vi "X410 ADC Read.vi"() -> (3 "Data out":T1[](array[typedef]))   [LabVIEW 2023]
uses:
  <instrlib>/_niInstr/DSP/v1/Shared/Public/IQ Data.ctl
  <vilib>/rvi/eio/common/nirviEmuTemplateMethod_errors.vi
  <instrlib>/_niInstr/DSP/v1/FPGA/Public/Sub VIs/Data Conversion/I16 to IQ - 1 spc - S18.1.vi
  <vilib>/eio/EIONode/EIONode.xnode
  <instrlib>/_niInstr/DSP/v1/FPGA/niInstr DSP v1 FPGA.lvlib
  <instrlib>/_niInstr/DSP/v1/Shared/niInstr DSP v1 Shared.lvlib
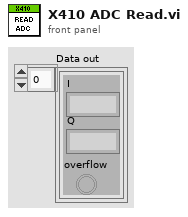
[diagram p1: front panel]
types:
  T1 = typedef "niInstr DSP v1 Shared.lvlib/IQ Data.ctl" = cluster{"I":fxp<+/-,18,1>, "Q":fxp<+/-,18,1>, "overflow":bool}
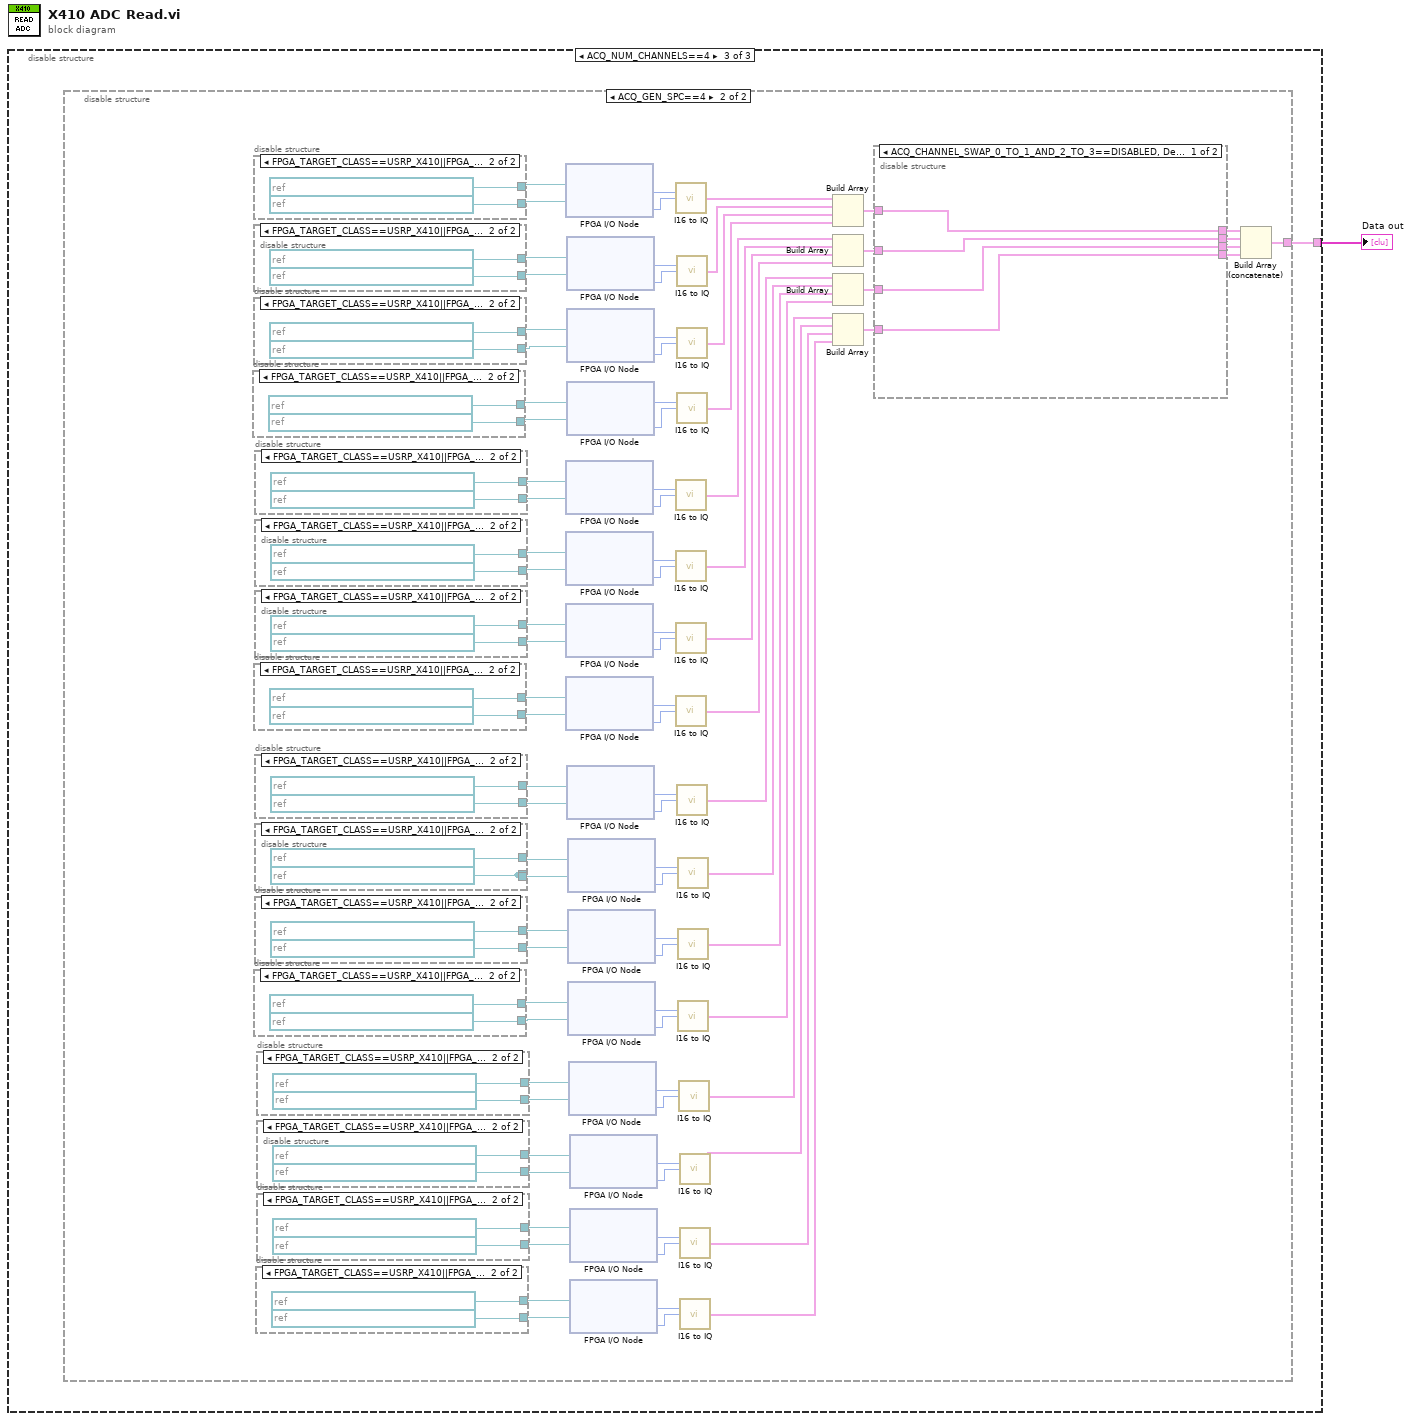
[diagram p0: block diagram]
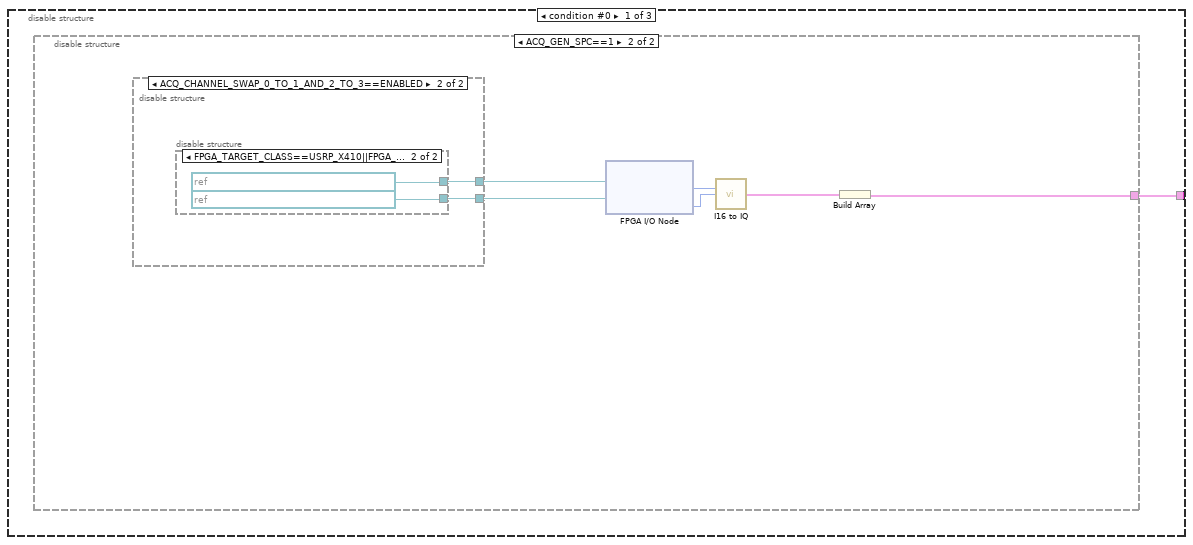
[diagram p2: hidden frame]
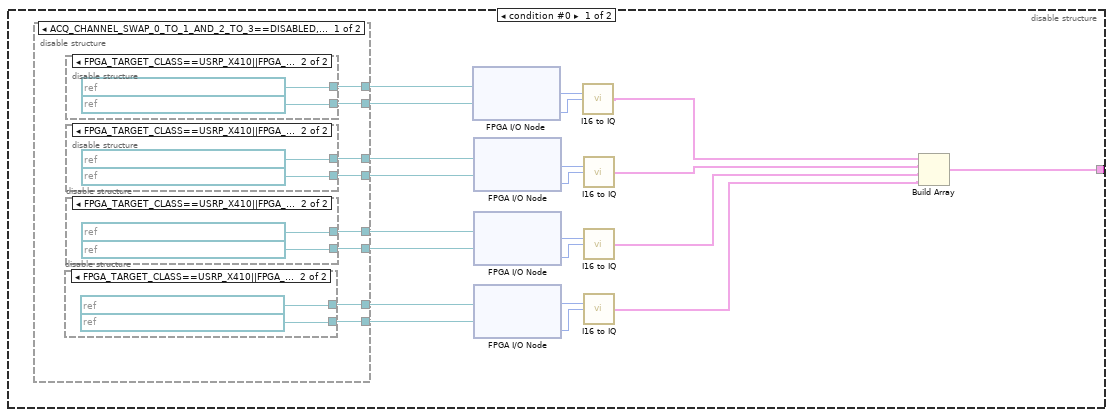
[diagram p3: hidden frame]
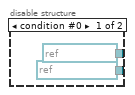
[diagram p4: hidden frame]
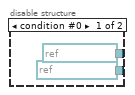
[diagram p5: hidden frame]
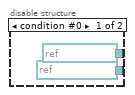
[diagram p6: hidden frame]
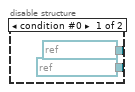
[diagram p7: hidden frame]
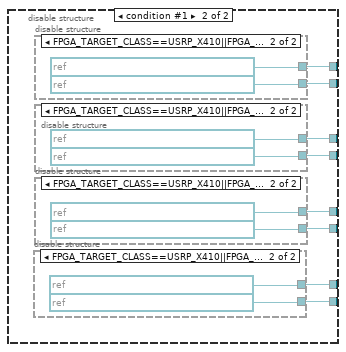
[diagram p8: hidden frame]
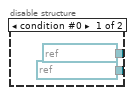
[diagram p9: hidden frame]
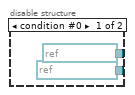
[diagram p10: hidden frame]
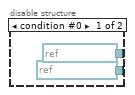
[diagram p11: hidden frame]
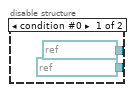
[diagram p12: hidden frame]
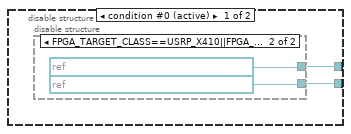
[diagram p13: hidden frame]
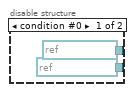
[diagram p14: hidden frame]
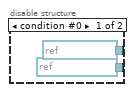
[diagram p15: hidden frame]
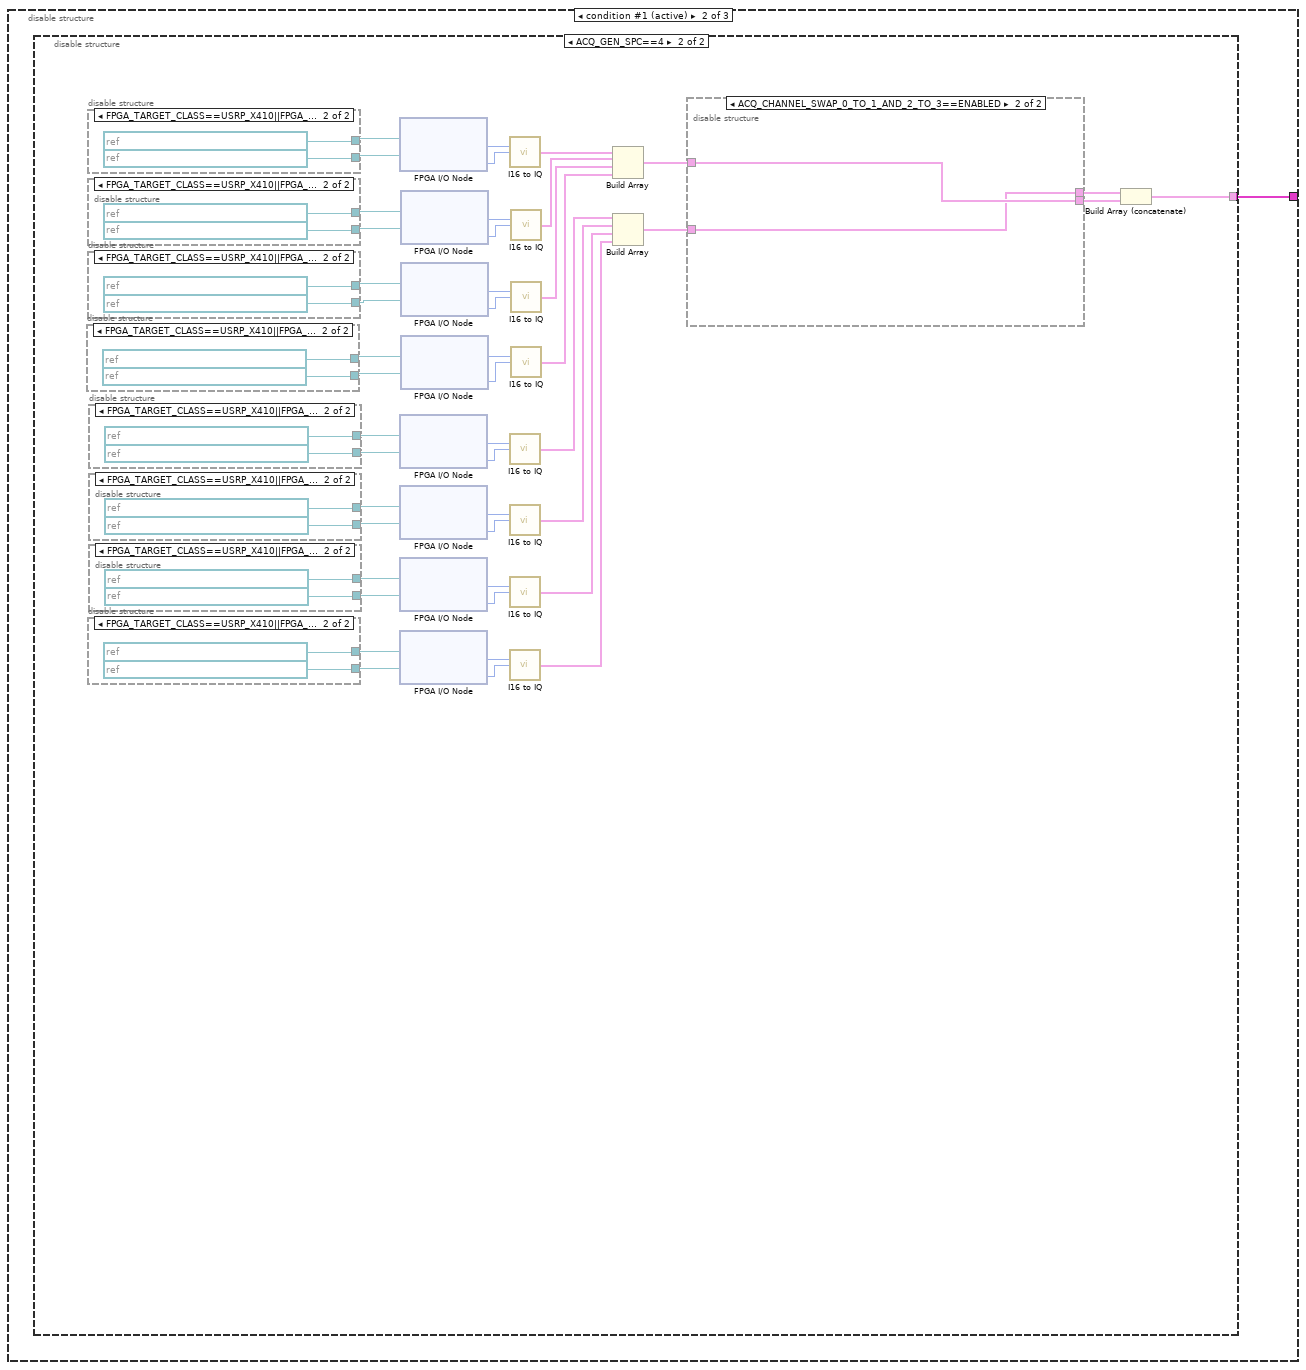
[diagram p16: hidden frame]
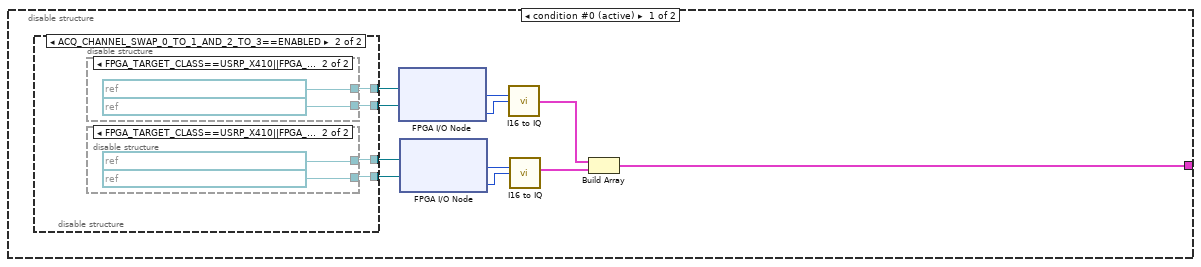
[diagram p17: hidden frame]
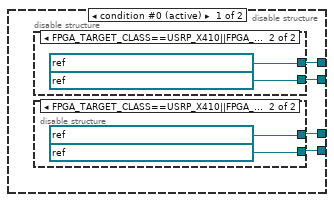
[diagram p18: hidden frame]
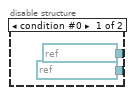
[diagram p19: hidden frame]
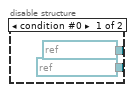
[diagram p20: hidden frame]
diagram:
  n1 = disable-structure shown="ACQ_NUM_CHANNELS==4" {
    disable-tunnel: [w2 w90 w207] -> w1
    frame condition #0 {
      n2 = disable-structure shown="ACQ_GEN_SPC==1" {
        disable-tunnel: [w15 w77] -> w2
        frame condition #0 {
          n3 = disable-structure shown="ACQ_CHANNEL_SWAP_0_TO_1_AND_2_TO_3==DISABLED, Default" {
            disable-tunnel: [w31 w55] -> w10
            disable-tunnel: [w30 w54] -> w9
            disable-tunnel: [w29 w53] -> w8
            disable-tunnel: [w28 w52] -> w7
            disable-tunnel: [w27 w51] -> w6
            disable-tunnel: [w26 w50] -> w5
            disable-tunnel: [w25 w49] -> w4
            disable-tunnel: [w24 w48] -> w3
            frame condition #0 (active) {
              n4 = disable-structure shown="FPGA_TARGET_CLASS==USRP_X410||FPGA_TARGET_CLASS==USRP_X410__EMBEDDED____UNSUPPORTED" {
                disable-tunnel: [refnum<k21> "RF 0/Rx/Q" ("FPGA I/O In") refnum<k21> "Daughterboard 0\\RF 0.Rx.Q3" ("FPGA I/O In")] -> w24
                disable-tunnel: [refnum<k21> "RF 0/Rx/I" ("FPGA I/O In") refnum<k21> "Daughterboard 0\\RF 0.Rx.I3" ("FPGA I/O In")] -> w25
                frame condition #0 {
                }
                frame condition #1 (active) {
                }
              }
              n5 = disable-structure shown="FPGA_TARGET_CLASS==USRP_X410||FPGA_TARGET_CLASS==USRP_X410__EMBEDDED____UNSUPPORTED" {
                disable-tunnel: [refnum<k21> "RF 0/Rx/Q" ("FPGA I/O In") refnum<k21> "Daughterboard 0\\RF 0.Rx.Q0" ("FPGA I/O In")] -> w30
                disable-tunnel: [refnum<k21> "RF 0/Rx/I" ("FPGA I/O In") refnum<k21> "Daughterboard 0\\RF 0.Rx.I0" ("FPGA I/O In")] -> w31
                frame condition #0 {
                }
                frame condition #1 (active) {
                }
              }
              n6 = disable-structure shown="FPGA_TARGET_CLASS==USRP_X410||FPGA_TARGET_CLASS==USRP_X410__EMBEDDED____UNSUPPORTED" {
                disable-tunnel: [refnum<k21> "RF 0/Rx/Q" ("FPGA I/O In") refnum<k21> "Daughterboard 0\\RF 0.Rx.Q1" ("FPGA I/O In")] -> w28
                disable-tunnel: [refnum<k21> "RF 0/Rx/I" ("FPGA I/O In") refnum<k21> "Daughterboard 0\\RF 0.Rx.I1" ("FPGA I/O In")] -> w29
                frame condition #0 {
                }
                frame condition #1 (active) {
                }
              }
              n7 = disable-structure shown="FPGA_TARGET_CLASS==USRP_X410||FPGA_TARGET_CLASS==USRP_X410__EMBEDDED____UNSUPPORTED" {
                disable-tunnel: [refnum<k21> "RF 0/Rx/Q" ("FPGA I/O In") refnum<k21> "Daughterboard 0\\RF 0.Rx.Q2" ("FPGA I/O In")] -> w26
                disable-tunnel: [refnum<k21> "RF 0/Rx/I" ("FPGA I/O In") refnum<k21> "Daughterboard 0\\RF 0.Rx.I2" ("FPGA I/O In")] -> w27
                frame condition #0 {
                }
                frame condition #1 (active) {
                }
              }
            }
            frame condition #1 {
              n8 = disable-structure shown="FPGA_TARGET_CLASS==USRP_X410||FPGA_TARGET_CLASS==USRP_X410__EMBEDDED____UNSUPPORTED" {
                disable-tunnel: [refnum<k21> "RF 0/Rx/Q" ("FPGA I/O In") refnum<k21> "Daughterboard 0\\Ch1RxDataQ3" ("FPGA I/O In")] -> w48
                disable-tunnel: [refnum<k21> "RF 0/Rx/I" ("FPGA I/O In") refnum<k21> "Daughterboard 0\\Ch1RxDataI3" ("FPGA I/O In")] -> w49
                frame condition #0 {
                }
                frame condition #1 (active) {
                }
              }
              n9 = disable-structure shown="FPGA_TARGET_CLASS==USRP_X410||FPGA_TARGET_CLASS==USRP_X410__EMBEDDED____UNSUPPORTED" {
                disable-tunnel: [refnum<k21> "RF 0/Rx/Q" ("FPGA I/O In") refnum<k21> "Daughterboard 0\\Ch1RxDataQ0" ("FPGA I/O In")] -> w54
                disable-tunnel: [refnum<k21> "RF 0/Rx/I" ("FPGA I/O In") refnum<k21> "Daughterboard 0\\Ch1RxDataI0" ("FPGA I/O In")] -> w55
                frame condition #0 {
                }
                frame condition #1 (active) {
                }
              }
              n10 = disable-structure shown="FPGA_TARGET_CLASS==USRP_X410||FPGA_TARGET_CLASS==USRP_X410__EMBEDDED____UNSUPPORTED" {
                disable-tunnel: [refnum<k21> "RF 0/Rx/Q" ("FPGA I/O In") refnum<k21> "Daughterboard 0\\Ch1RxDataQ1" ("FPGA I/O In")] -> w52
                disable-tunnel: [refnum<k21> "RF 0/Rx/I" ("FPGA I/O In") refnum<k21> "Daughterboard 0\\Ch1RxDataI1" ("FPGA I/O In")] -> w53
                frame condition #0 {
                }
                frame condition #1 (active) {
                }
              }
              n11 = disable-structure shown="FPGA_TARGET_CLASS==USRP_X410||FPGA_TARGET_CLASS==USRP_X410__EMBEDDED____UNSUPPORTED" {
                disable-tunnel: [refnum<k21> "RF 0/Rx/Q" ("FPGA I/O In") refnum<k21> "Daughterboard 0\\Ch1RxDataQ2" ("FPGA I/O In")] -> w50
                disable-tunnel: [refnum<k21> "RF 0/Rx/I" ("FPGA I/O In") refnum<k21> "Daughterboard 0\\Ch1RxDataI2" ("FPGA I/O In")] -> w51
                frame condition #0 {
                }
                frame condition #1 (active) {
                }
              }
            }
          }
          n12 = xnode "FPGA I/O Node"("FPGA I/O In"=w10, "FPGA I/O In"=w9) -> ("I/O Item"=w23:i16, "I/O Item"=w22:i16)  [unwired: 2 out]
          n13 = xnode "FPGA I/O Node"("FPGA I/O In"=w8, "FPGA I/O In"=w7) -> ("I/O Item"=w21:i16, "I/O Item"=w20:i16)  [unwired: 2 out]
          n14 = xnode "FPGA I/O Node"("FPGA I/O In"=w6, "FPGA I/O In"=w5) -> ("I/O Item"=w19:i16, "I/O Item"=w18:i16)  [unwired: 2 out]
          n15 = xnode "FPGA I/O Node"("FPGA I/O In"=w4, "FPGA I/O In"=w3) -> ("I/O Item"=w17:i16, "I/O Item"=w16:i16)  [unwired: 2 out]
          n16 = call-poly <instrlib>:"I16 to IQ.vi"("I"=w23, "Q"=w22) -> ("IQ"=w11:T1)  [unwired: 13 in]
          n17 = call-poly <instrlib>:"I16 to IQ.vi"("I"=w21, "Q"=w20) -> ("IQ"=w14:T1)  [unwired: 13 in]
          n18 = call-poly <instrlib>:"I16 to IQ.vi"("I"=w19, "Q"=w18) -> ("IQ"=w13:T1)  [unwired: 13 in]
          n19 = call-poly <instrlib>:"I16 to IQ.vi"("I"=w17, "Q"=w16) -> ("IQ"=w12:T1)  [unwired: 13 in]
          n20 = Build Array(w11, w14, w13, w12) -> (w15:T1[])
        }
        frame condition #1 (active) {
          n21 = disable-structure shown="ACQ_CHANNEL_SWAP_0_TO_1_AND_2_TO_3==ENABLED" {
            disable-tunnel: [w79 w85] -> w73
            disable-tunnel: [w78 w84] -> w72
            frame condition #0 (active) {
              n22 = disable-structure shown="FPGA_TARGET_CLASS==USRP_X410||FPGA_TARGET_CLASS==USRP_X410__EMBEDDED____UNSUPPORTED" {
                disable-tunnel: [refnum<k21> "RF 0/Rx/Q" ("FPGA I/O In") refnum<k21> "Daughterboard 0\\RF 0.Rx.Q" ("FPGA I/O In")] -> w78
                disable-tunnel: [refnum<k21> "RF 0/Rx/I" ("FPGA I/O In") refnum<k21> "Daughterboard 0\\RF 0.Rx.I" ("FPGA I/O In")] -> w79
                frame condition #0 {
                }
                frame condition #1 (active) {
                }
              }
            }
            frame condition #1 {
              n23 = disable-structure shown="FPGA_TARGET_CLASS==USRP_X410||FPGA_TARGET_CLASS==USRP_X410__EMBEDDED____UNSUPPORTED" {
                disable-tunnel: [refnum<k21> "RF 0/Rx/Q" ("FPGA I/O In") refnum<k21> "Daughterboard 0\\Ch1RxDataQ" ("FPGA I/O In")] -> w84
                disable-tunnel: [refnum<k21> "RF 0/Rx/I" ("FPGA I/O In") refnum<k21> "Daughterboard 0\\Ch1RxDataI" ("FPGA I/O In")] -> w85
                frame condition #0 {
                }
                frame condition #1 (active) {
                }
              }
            }
          }
          n24 = xnode "FPGA I/O Node"("FPGA I/O In"=w73, "FPGA I/O In"=w72) -> ("I/O Item"=w76:i16, "I/O Item"=w75:i16)  [unwired: 2 out]
          n25 = call-poly <instrlib>:"I16 to IQ.vi"("I"=w76, "Q"=w75) -> ("IQ"=w74:T1)  [unwired: 13 in]
          n26 = Build Array(w74) -> (w77:T1[])
        }
      }
    }
    frame condition #1 (active) {
      n27 = disable-structure shown="ACQ_GEN_SPC==4" {
        disable-tunnel: [w91 w170] -> w90
        frame condition #0 (active) {
          n28 = disable-structure shown="ACQ_CHANNEL_SWAP_0_TO_1_AND_2_TO_3==ENABLED" {
            disable-tunnel: [w105 w117] -> w97
            disable-tunnel: [w104 w116] -> w96
            disable-tunnel: [w103 w115] -> w95
            disable-tunnel: [w102 w114] -> w94
            frame condition #0 (active) {
              n29 = disable-structure shown="FPGA_TARGET_CLASS==USRP_X410||FPGA_TARGET_CLASS==USRP_X410__EMBEDDED____UNSUPPORTED" {
                disable-tunnel: [refnum<k21> "RF 0/Rx/Q" ("FPGA I/O In") refnum<k21> "Daughterboard 0\\RF 0.Rx.Q" ("FPGA I/O In")] -> w103
                disable-tunnel: [refnum<k21> "RF 0/Rx/I" ("FPGA I/O In") refnum<k21> "Daughterboard 0\\RF 0.Rx.I" ("FPGA I/O In")] -> w102
                frame condition #0 {
                }
                frame condition #1 (active) {
                }
              }
              n30 = disable-structure shown="FPGA_TARGET_CLASS==USRP_X410||FPGA_TARGET_CLASS==USRP_X410__EMBEDDED____UNSUPPORTED" {
                disable-tunnel: [refnum<k21> "RF 0/Rx/Q" ("FPGA I/O In") refnum<k21> "Daughterboard 0\\RF 1.Rx.Q" ("FPGA I/O In")] -> w105
                disable-tunnel: [refnum<k21> "RF 0/Rx/I" ("FPGA I/O In") refnum<k21> "Daughterboard 0\\RF 1.Rx.I" ("FPGA I/O In")] -> w104
                frame condition #0 {
                }
                frame condition #1 (active) {
                }
              }
            }
            frame condition #1 {
              n31 = disable-structure shown="FPGA_TARGET_CLASS==USRP_X410||FPGA_TARGET_CLASS==USRP_X410__EMBEDDED____UNSUPPORTED" {
                disable-tunnel: [refnum<k21> "RF 0/Rx/Q" ("FPGA I/O In") refnum<k21> "Daughterboard 0\\Ch1RxDataQ" ("FPGA I/O In")] -> w115
                disable-tunnel: [refnum<k21> "RF 0/Rx/I" ("FPGA I/O In") refnum<k21> "Daughterboard 0\\Ch1RxDataI" ("FPGA I/O In")] -> w114
                frame condition #0 {
                }
                frame condition #1 (active) {
                }
              }
              n32 = disable-structure shown="FPGA_TARGET_CLASS==USRP_X410||FPGA_TARGET_CLASS==USRP_X410__EMBEDDED____UNSUPPORTED" {
                disable-tunnel: [refnum<k21> "RF 0/Rx/Q" ("FPGA I/O In") refnum<k21> "Daughterboard 0\\Ch0RxDataQ" ("FPGA I/O In")] -> w117
                disable-tunnel: [refnum<k21> "RF 0/Rx/I" ("FPGA I/O In") refnum<k21> "Daughterboard 0\\Ch0RxDataI" ("FPGA I/O In")] -> w116
                frame condition #0 {
                }
                frame condition #1 (active) {
                }
              }
            }
          }
          n33 = xnode "FPGA I/O Node"("FPGA I/O In"=w94, "FPGA I/O In"=w95) -> ("I/O Item"=w101:i16, "I/O Item"=w100:i16)  [unwired: 2 out]
          n34 = xnode "FPGA I/O Node"("FPGA I/O In"=w96, "FPGA I/O In"=w97) -> ("I/O Item"=w99:i16, "I/O Item"=w98:i16)  [unwired: 2 out]
          n35 = call-poly <instrlib>:"I16 to IQ.vi"("I"=w101, "Q"=w100) -> ("IQ"=w93:T1)  [unwired: 13 in]
          n36 = call-poly <instrlib>:"I16 to IQ.vi"("I"=w99, "Q"=w98) -> ("IQ"=w92:T1)  [unwired: 13 in]
          n37 = Build Array(w93, w92) -> (w91:T1[])
        }
        frame condition #1 {
          n38 = disable-structure shown="FPGA_TARGET_CLASS==USRP_X410||FPGA_TARGET_CLASS==USRP_X410__EMBEDDED____UNSUPPORTED" {
            disable-tunnel: [refnum<k21> "RF 0/Rx/Q" ("FPGA I/O In") refnum<k21> "Daughterboard 0\\RF 0.Rx.Q3" ("FPGA I/O In")] -> w145
            disable-tunnel: [refnum<k21> "RF 0/Rx/I" ("FPGA I/O In") refnum<k21> "Daughterboard 0\\RF 0.Rx.I3" ("FPGA I/O In")] -> w144
            frame condition #0 {
            }
            frame condition #1 (active) {
            }
          }
          n39 = disable-structure shown="FPGA_TARGET_CLASS==USRP_X410||FPGA_TARGET_CLASS==USRP_X410__EMBEDDED____UNSUPPORTED" {
            disable-tunnel: [refnum<k21> "RF 0/Rx/Q" ("FPGA I/O In") refnum<k21> "Daughterboard 0\\RF 0.Rx.Q0" ("FPGA I/O In")] -> w139
            disable-tunnel: [refnum<k21> "RF 0/Rx/I" ("FPGA I/O In") refnum<k21> "Daughterboard 0\\RF 0.Rx.I0" ("FPGA I/O In")] -> w138
            frame condition #0 {
            }
            frame condition #1 (active) {
            }
          }
          n40 = disable-structure shown="FPGA_TARGET_CLASS==USRP_X410||FPGA_TARGET_CLASS==USRP_X410__EMBEDDED____UNSUPPORTED" {
            disable-tunnel: [refnum<k21> "RF 0/Rx/Q" ("FPGA I/O In") refnum<k21> "Daughterboard 0\\RF 0.Rx.Q1" ("FPGA I/O In")] -> w141
            disable-tunnel: [refnum<k21> "RF 0/Rx/I" ("FPGA I/O In") refnum<k21> "Daughterboard 0\\RF 0.Rx.I1" ("FPGA I/O In")] -> w140
            frame condition #0 {
            }
            frame condition #1 (active) {
            }
          }
          n41 = disable-structure shown="FPGA_TARGET_CLASS==USRP_X410||FPGA_TARGET_CLASS==USRP_X410__EMBEDDED____UNSUPPORTED" {
            disable-tunnel: [refnum<k21> "RF 0/Rx/Q" ("FPGA I/O In") refnum<k21> "Daughterboard 0\\RF 0.Rx.Q2" ("FPGA I/O In")] -> w143
            disable-tunnel: [refnum<k21> "RF 0/Rx/I" ("FPGA I/O In") refnum<k21> "Daughterboard 0\\RF 0.Rx.I2" ("FPGA I/O In")] -> w142
            frame condition #0 {
            }
            frame condition #1 (active) {
            }
          }
          n42 = disable-structure shown="FPGA_TARGET_CLASS==USRP_X410||FPGA_TARGET_CLASS==USRP_X410__EMBEDDED____UNSUPPORTED" {
            disable-tunnel: [refnum<k21> "RF 0/Rx/Q" ("FPGA I/O In") refnum<k21> "Daughterboard 0\\RF 1.Rx.Q3" ("FPGA I/O In")] -> w153
            disable-tunnel: [refnum<k21> "RF 0/Rx/I" ("FPGA I/O In") refnum<k21> "Daughterboard 0\\RF 1.Rx.I3" ("FPGA I/O In")] -> w152
            frame condition #0 {
            }
            frame condition #1 (active) {
            }
          }
          n43 = disable-structure shown="FPGA_TARGET_CLASS==USRP_X410||FPGA_TARGET_CLASS==USRP_X410__EMBEDDED____UNSUPPORTED" {
            disable-tunnel: [refnum<k21> "RF 0/Rx/Q" ("FPGA I/O In") refnum<k21> "Daughterboard 0\\RF 1.Rx.Q0" ("FPGA I/O In")] -> w147
            disable-tunnel: [refnum<k21> "RF 0/Rx/I" ("FPGA I/O In") refnum<k21> "Daughterboard 0\\RF 1.Rx.I0" ("FPGA I/O In")] -> w146
            frame condition #0 {
            }
            frame condition #1 (active) {
            }
          }
          n44 = disable-structure shown="FPGA_TARGET_CLASS==USRP_X410||FPGA_TARGET_CLASS==USRP_X410__EMBEDDED____UNSUPPORTED" {
            disable-tunnel: [refnum<k21> "RF 0/Rx/Q" ("FPGA I/O In") refnum<k21> "Daughterboard 0\\RF 1.Rx.Q1" ("FPGA I/O In")] -> w149
            disable-tunnel: [refnum<k21> "RF 0/Rx/I" ("FPGA I/O In") refnum<k21> "Daughterboard 0\\RF 1.Rx.I1" ("FPGA I/O In")] -> w148
            frame condition #0 {
            }
            frame condition #1 (active) {
            }
          }
          n45 = disable-structure shown="FPGA_TARGET_CLASS==USRP_X410||FPGA_TARGET_CLASS==USRP_X410__EMBEDDED____UNSUPPORTED" {
            disable-tunnel: [refnum<k21> "RF 0/Rx/Q" ("FPGA I/O In") refnum<k21> "Daughterboard 0\\RF 1.Rx.Q2" ("FPGA I/O In")] -> w151
            disable-tunnel: [refnum<k21> "RF 0/Rx/I" ("FPGA I/O In") refnum<k21> "Daughterboard 0\\RF 1.Rx.I2" ("FPGA I/O In")] -> w150
            frame condition #0 {
            }
            frame condition #1 (active) {
            }
          }
          n46 = xnode "FPGA I/O Node"("FPGA I/O In"=w138, "FPGA I/O In"=w139) -> ("I/O Item"=w169:i16, "I/O Item"=w168:i16)  [unwired: 2 out]
          n47 = xnode "FPGA I/O Node"("FPGA I/O In"=w146, "FPGA I/O In"=w147) -> ("I/O Item"=w161:i16, "I/O Item"=w160:i16)  [unwired: 2 out]
          n48 = xnode "FPGA I/O Node"("FPGA I/O In"=w148, "FPGA I/O In"=w149) -> ("I/O Item"=w159:i16, "I/O Item"=w158:i16)  [unwired: 2 out]
          n49 = xnode "FPGA I/O Node"("FPGA I/O In"=w150, "FPGA I/O In"=w151) -> ("I/O Item"=w157:i16, "I/O Item"=w156:i16)  [unwired: 2 out]
          n50 = xnode "FPGA I/O Node"("FPGA I/O In"=w152, "FPGA I/O In"=w153) -> ("I/O Item"=w155:i16, "I/O Item"=w154:i16)  [unwired: 2 out]
          n51 = xnode "FPGA I/O Node"("FPGA I/O In"=w140, "FPGA I/O In"=w141) -> ("I/O Item"=w167:i16, "I/O Item"=w166:i16)  [unwired: 2 out]
          n52 = xnode "FPGA I/O Node"("FPGA I/O In"=w142, "FPGA I/O In"=w143) -> ("I/O Item"=w165:i16, "I/O Item"=w164:i16)  [unwired: 2 out]
          n53 = xnode "FPGA I/O Node"("FPGA I/O In"=w144, "FPGA I/O In"=w145) -> ("I/O Item"=w163:i16, "I/O Item"=w162:i16)  [unwired: 2 out]
          n54 = call-poly <instrlib>:"I16 to IQ.vi"("I"=w169, "Q"=w168) -> ("IQ"=w137:T1)  [unwired: 13 in]
          n55 = call-poly <instrlib>:"I16 to IQ.vi"("I"=w161, "Q"=w160) -> ("IQ"=w133:T1)  [unwired: 13 in]
          n56 = call-poly <instrlib>:"I16 to IQ.vi"("I"=w159, "Q"=w158) -> ("IQ"=w132:T1)  [unwired: 13 in]
          n57 = call-poly <instrlib>:"I16 to IQ.vi"("I"=w157, "Q"=w156) -> ("IQ"=w131:T1)  [unwired: 13 in]
          n58 = call-poly <instrlib>:"I16 to IQ.vi"("I"=w155, "Q"=w154) -> ("IQ"=w130:T1)  [unwired: 13 in]
          n59 = call-poly <instrlib>:"I16 to IQ.vi"("I"=w167, "Q"=w166) -> ("IQ"=w136:T1)  [unwired: 13 in]
          n60 = call-poly <instrlib>:"I16 to IQ.vi"("I"=w165, "Q"=w164) -> ("IQ"=w135:T1)  [unwired: 13 in]
          n61 = call-poly <instrlib>:"I16 to IQ.vi"("I"=w163, "Q"=w162) -> ("IQ"=w134:T1)  [unwired: 13 in]
          n62 = Build Array(w137, w136, w135, w134) -> (w129:T1[])
          n63 = Build Array(w133, w132, w131, w130) -> (w127:T1[])
          n64 = disable-structure shown="ACQ_CHANNEL_SWAP_0_TO_1_AND_2_TO_3==ENABLED" {
            disable-tunnel: w129 -> [w172 w174]
            disable-tunnel: [w172 w173] -> w128
            disable-tunnel: [w171 w174] -> w126
            disable-tunnel: w127 -> [w171 w173]
            frame condition #0 (active) {
            }
            frame condition #1 {
            }
          }
          n65 = Build Array (concatenate)(w128, w126) -> (w170:T1[])
        }
      }
    }
    frame condition #2 {
      n66 = disable-structure shown="ACQ_GEN_SPC==4" {
        disable-tunnel: [w216 w345] -> w207
        frame condition #0 (active) {
          n67 = disable-structure shown="FPGA_TARGET_CLASS==USRP_X410||FPGA_TARGET_CLASS==USRP_X410__EMBEDDED____UNSUPPORTED" {
            disable-tunnel: [refnum<k21> "RF 0/Rx/Q" ("FPGA I/O In") refnum<k21> "Daughterboard 1\\RF 1.Rx.Q" ("FPGA I/O In")] -> w224
            disable-tunnel: [refnum<k21> "RF 0/Rx/I" ("FPGA I/O In") refnum<k21> "Daughterboard 1\\RF 1.Rx.I" ("FPGA I/O In")] -> w223
            frame condition #0 {
            }
            frame condition #1 (active) {
            }
          }
          n68 = disable-structure shown="FPGA_TARGET_CLASS==USRP_X410||FPGA_TARGET_CLASS==USRP_X410__EMBEDDED____UNSUPPORTED" {
            disable-tunnel: [refnum<k21> "RF 0/Rx/Q" ("FPGA I/O In") refnum<k21> "Daughterboard 0\\RF 0.Rx.Q" ("FPGA I/O In")] -> w218
            disable-tunnel: [refnum<k21> "RF 0/Rx/I" ("FPGA I/O In") refnum<k21> "Daughterboard 0\\RF 0.Rx.I" ("FPGA I/O In")] -> w217
            frame condition #0 {
            }
            frame condition #1 (active) {
            }
          }
          n69 = disable-structure shown="FPGA_TARGET_CLASS==USRP_X410||FPGA_TARGET_CLASS==USRP_X410__EMBEDDED____UNSUPPORTED" {
            disable-tunnel: [refnum<k21> "RF 0/Rx/Q" ("FPGA I/O In") refnum<k21> "Daughterboard 0\\RF 1.Rx.Q" ("FPGA I/O In")] -> w220
            disable-tunnel: [refnum<k21> "RF 0/Rx/I" ("FPGA I/O In") refnum<k21> "Daughterboard 0\\RF 1.Rx.I" ("FPGA I/O In")] -> w219
            frame condition #0 {
            }
            frame condition #1 (active) {
            }
          }
          n70 = disable-structure shown="FPGA_TARGET_CLASS==USRP_X410||FPGA_TARGET_CLASS==USRP_X410__EMBEDDED____UNSUPPORTED" {
            disable-tunnel: [refnum<k21> "RF 0/Rx/Q" ("FPGA I/O In") refnum<k21> "Daughterboard 1\\RF 0.Rx.Q" ("FPGA I/O In")] -> w222
            disable-tunnel: [refnum<k21> "RF 0/Rx/I" ("FPGA I/O In") refnum<k21> "Daughterboard 1\\RF 0.Rx.I" ("FPGA I/O In")] -> w221
            frame condition #0 {
            }
            frame condition #1 (active) {
            }
          }
          n71 = xnode "FPGA I/O Node"("FPGA I/O In"=w217, "FPGA I/O In"=w218) -> ("I/O Item"=w232:i16, "I/O Item"=w231:i16)  [unwired: 2 out]
          n72 = xnode "FPGA I/O Node"("FPGA I/O In"=w219, "FPGA I/O In"=w220) -> ("I/O Item"=w230:i16, "I/O Item"=w229:i16)  [unwired: 2 out]
          n73 = xnode "FPGA I/O Node"("FPGA I/O In"=w221, "FPGA I/O In"=w222) -> ("I/O Item"=w228:i16, "I/O Item"=w227:i16)  [unwired: 2 out]
          n74 = xnode "FPGA I/O Node"("FPGA I/O In"=w223, "FPGA I/O In"=w224) -> ("I/O Item"=w226:i16, "I/O Item"=w225:i16)  [unwired: 2 out]
          n75 = call-poly <instrlib>:"I16 to IQ.vi"("I"=w232, "Q"=w231) -> ("IQ"=w215:T1)  [unwired: 13 in]
          n76 = call-poly <instrlib>:"I16 to IQ.vi"("I"=w230, "Q"=w229) -> ("IQ"=w210:T1)  [unwired: 13 in]
          n77 = call-poly <instrlib>:"I16 to IQ.vi"("I"=w228, "Q"=w227) -> ("IQ"=w209:T1)  [unwired: 13 in]
          n78 = call-poly <instrlib>:"I16 to IQ.vi"("I"=w226, "Q"=w225) -> ("IQ"=w208:T1)  [unwired: 13 in]
          n79 = disable-structure shown="ACQ_CHANNEL_SWAP_0_TO_1_AND_2_TO_3==ENABLED" {
            disable-tunnel: w215 -> [w235 w239]
            disable-tunnel: [w236 w239] -> w213
            disable-tunnel: w210 -> [w236 w240]
            disable-tunnel: [w235 w240] -> w214
            disable-tunnel: [w234 w238] -> w212
            disable-tunnel: w209 -> [w234 w237]
            disable-tunnel: [w233 w237] -> w211
            disable-tunnel: w208 -> [w233 w238]
            frame condition #0 (active) {
            }
            frame condition #1 {
            }
          }
          n80 = Build Array(w214, w213, w212, w211) -> (w216:T1[])
        }
        frame condition #1 {
          n81 = disable-structure shown="FPGA_TARGET_CLASS==USRP_X410||FPGA_TARGET_CLASS==USRP_X410__EMBEDDED____UNSUPPORTED" {
            disable-tunnel: [refnum<k21> "RF 0/Rx/Q" ("FPGA I/O In") refnum<k21> "Daughterboard 0\\RF 0.Rx.Q3" ("FPGA I/O In")] -> w288
            disable-tunnel: [refnum<k21> "RF 0/Rx/I" ("FPGA I/O In") refnum<k21> "Daughterboard 0\\RF 0.Rx.I3" ("FPGA I/O In")] -> w287
            frame condition #0 {
            }
            frame condition #1 (active) {
            }
          }
          n82 = disable-structure shown="FPGA_TARGET_CLASS==USRP_X410||FPGA_TARGET_CLASS==USRP_X410__EMBEDDED____UNSUPPORTED" {
            disable-tunnel: [refnum<k21> "RF 0/Rx/Q" ("FPGA I/O In") refnum<k21> "Daughterboard 0\\RF 0.Rx.Q0" ("FPGA I/O In")] -> w282
            disable-tunnel: [refnum<k21> "RF 0/Rx/I" ("FPGA I/O In") refnum<k21> "Daughterboard 0\\RF 0.Rx.I0" ("FPGA I/O In")] -> w281
            frame condition #0 {
            }
            frame condition #1 (active) {
            }
          }
          n83 = disable-structure shown="FPGA_TARGET_CLASS==USRP_X410||FPGA_TARGET_CLASS==USRP_X410__EMBEDDED____UNSUPPORTED" {
            disable-tunnel: [refnum<k21> "RF 0/Rx/Q" ("FPGA I/O In") refnum<k21> "Daughterboard 0\\RF 0.Rx.Q1" ("FPGA I/O In")] -> w284
            disable-tunnel: [refnum<k21> "RF 0/Rx/I" ("FPGA I/O In") refnum<k21> "Daughterboard 0\\RF 0.Rx.I1" ("FPGA I/O In")] -> w283
            frame condition #0 {
            }
            frame condition #1 (active) {
            }
          }
          n84 = disable-structure shown="FPGA_TARGET_CLASS==USRP_X410||FPGA_TARGET_CLASS==USRP_X410__EMBEDDED____UNSUPPORTED" {
            disable-tunnel: [refnum<k21> "RF 0/Rx/Q" ("FPGA I/O In") refnum<k21> "Daughterboard 0\\RF 0.Rx.Q2" ("FPGA I/O In")] -> w286
            disable-tunnel: [refnum<k21> "RF 0/Rx/I" ("FPGA I/O In") refnum<k21> "Daughterboard 0\\RF 0.Rx.I2" ("FPGA I/O In")] -> w285
            frame condition #0 {
            }
            frame condition #1 (active) {
            }
          }
          n85 = disable-structure shown="FPGA_TARGET_CLASS==USRP_X410||FPGA_TARGET_CLASS==USRP_X410__EMBEDDED____UNSUPPORTED" {
            disable-tunnel: [refnum<k21> "RF 0/Rx/Q" ("FPGA I/O In") refnum<k21> "Daughterboard 0\\RF 1.Rx.Q3" ("FPGA I/O In")] -> w296
            disable-tunnel: [refnum<k21> "RF 0/Rx/I" ("FPGA I/O In") refnum<k21> "Daughterboard 0\\RF 1.Rx.I3" ("FPGA I/O In")] -> w295
            frame condition #0 {
            }
            frame condition #1 (active) {
            }
          }
          n86 = disable-structure shown="FPGA_TARGET_CLASS==USRP_X410||FPGA_TARGET_CLASS==USRP_X410__EMBEDDED____UNSUPPORTED" {
            disable-tunnel: [refnum<k21> "RF 0/Rx/Q" ("FPGA I/O In") refnum<k21> "Daughterboard 1\\RF 0.Rx.Q3" ("FPGA I/O In")] -> w304
            disable-tunnel: [refnum<k21> "RF 0/Rx/I" ("FPGA I/O In") refnum<k21> "Daughterboard 1\\RF 0.Rx.I3" ("FPGA I/O In")] -> w303
            frame condition #0 {
            }
            frame condition #1 (active) {
            }
          }
          n87 = disable-structure shown="FPGA_TARGET_CLASS==USRP_X410||FPGA_TARGET_CLASS==USRP_X410__EMBEDDED____UNSUPPORTED" {
            disable-tunnel: [refnum<k21> "RF 0/Rx/Q" ("FPGA I/O In") refnum<k21> "Daughterboard 0\\RF 1.Rx.Q0" ("FPGA I/O In")] -> w290
            disable-tunnel: [refnum<k21> "RF 0/Rx/I" ("FPGA I/O In") refnum<k21> "Daughterboard 0\\RF 1.Rx.I0" ("FPGA I/O In")] -> w289
            frame condition #0 {
            }
            frame condition #1 (active) {
            }
          }
          n88 = disable-structure shown="FPGA_TARGET_CLASS==USRP_X410||FPGA_TARGET_CLASS==USRP_X410__EMBEDDED____UNSUPPORTED" {
            disable-tunnel: [refnum<k21> "RF 0/Rx/Q" ("FPGA I/O In") refnum<k21> "Daughterboard 0\\RF 1.Rx.Q1" ("FPGA I/O In")] -> w292
            disable-tunnel: [refnum<k21> "RF 0/Rx/I" ("FPGA I/O In") refnum<k21> "Daughterboard 0\\RF 1.Rx.I1" ("FPGA I/O In")] -> w291
            frame condition #0 {
            }
            frame condition #1 (active) {
            }
          }
          n89 = disable-structure shown="FPGA_TARGET_CLASS==USRP_X410||FPGA_TARGET_CLASS==USRP_X410__EMBEDDED____UNSUPPORTED" {
            disable-tunnel: [refnum<k21> "RF 0/Rx/Q" ("FPGA I/O In") refnum<k21> "Daughterboard 0\\RF 1.Rx.Q2" ("FPGA I/O In")] -> w294
            disable-tunnel: [refnum<k21> "RF 0/Rx/I" ("FPGA I/O In") refnum<k21> "Daughterboard 0\\RF 1.Rx.I2" ("FPGA I/O In")] -> w293
            frame condition #0 {
            }
            frame condition #1 (active) {
            }
          }
          n90 = disable-structure shown="FPGA_TARGET_CLASS==USRP_X410||FPGA_TARGET_CLASS==USRP_X410__EMBEDDED____UNSUPPORTED" {
            disable-tunnel: [refnum<k21> "RF 0/Rx/Q" ("FPGA I/O In") refnum<k21> "Daughterboard 1\\RF 0.Rx.Q0" ("FPGA I/O In")] -> w298
            disable-tunnel: [refnum<k21> "RF 0/Rx/I" ("FPGA I/O In") refnum<k21> "Daughterboard 1\\RF 0.Rx.I0" ("FPGA I/O In")] -> w297
            frame condition #0 {
            }
            frame condition #1 (active) {
            }
          }
          n91 = disable-structure shown="FPGA_TARGET_CLASS==USRP_X410||FPGA_TARGET_CLASS==USRP_X410__EMBEDDED____UNSUPPORTED" {
            disable-tunnel: [refnum<k21> "RF 0/Rx/Q" ("FPGA I/O In") w380] -> _
            disable-tunnel: [refnum<k21> "RF 0/Rx/I" ("FPGA I/O In") refnum<k21> "Daughterboard 1\\RF 0.Rx.I1" ("FPGA I/O In")] -> w299
            disable-tunnel: [_ w380] -> w300
            frame condition #0 {
            }
            frame condition #1 (active) {
              w380 = refnum<k21> "Daughterboard 1\\RF 0.Rx.Q1" ("FPGA I/O In")
            }
          }
          n92 = disable-structure shown="FPGA_TARGET_CLASS==USRP_X410||FPGA_TARGET_CLASS==USRP_X410__EMBEDDED____UNSUPPORTED" {
            disable-tunnel: [refnum<k21> "RF 0/Rx/Q" ("FPGA I/O In") refnum<k21> "Daughterboard 1\\RF 0.Rx.Q2" ("FPGA I/O In")] -> w302
            disable-tunnel: [refnum<k21> "RF 0/Rx/I" ("FPGA I/O In") refnum<k21> "Daughterboard 1\\RF 0.Rx.I2" ("FPGA I/O In")] -> w301
            frame condition #0 {
            }
            frame condition #1 (active) {
            }
          }
          n93 = disable-structure shown="FPGA_TARGET_CLASS==USRP_X410||FPGA_TARGET_CLASS==USRP_X410__EMBEDDED____UNSUPPORTED" {
            disable-tunnel: [refnum<k21> "RF 0/Rx/Q" ("FPGA I/O In") refnum<k21> "Daughterboard 1\\RF 1.Rx.Q3" ("FPGA I/O In")] -> w309
            disable-tunnel: [refnum<k21> "RF 0/Rx/I" ("FPGA I/O In") refnum<k21> "Daughterboard 1\\RF 1.Rx.I3" ("FPGA I/O In")] -> w313
            frame condition #0 {
            }
            frame condition #1 (active) {
            }
          }
          n94 = disable-structure shown="FPGA_TARGET_CLASS==USRP_X410||FPGA_TARGET_CLASS==USRP_X410__EMBEDDED____UNSUPPORTED" {
            disable-tunnel: [refnum<k21> "RF 0/Rx/Q" ("FPGA I/O In") refnum<k21> "Daughterboard 1\\RF 1.Rx.Q0" ("FPGA I/O In")] -> w305
            disable-tunnel: [refnum<k21> "RF 0/Rx/I" ("FPGA I/O In") refnum<k21> "Daughterboard 1\\RF 1.Rx.I0" ("FPGA I/O In")] -> w306
            frame condition #0 {
            }
            frame condition #1 (active) {
            }
          }
          n95 = disable-structure shown="FPGA_TARGET_CLASS==USRP_X410||FPGA_TARGET_CLASS==USRP_X410__EMBEDDED____UNSUPPORTED" {
            disable-tunnel: [refnum<k21> "RF 0/Rx/Q" ("FPGA I/O In") refnum<k21> "Daughterboard 1\\RF 1.Rx.Q1" ("FPGA I/O In")] -> w308
            disable-tunnel: [refnum<k21> "RF 0/Rx/I" ("FPGA I/O In") refnum<k21> "Daughterboard 1\\RF 1.Rx.I1" ("FPGA I/O In")] -> w307
            frame condition #0 {
            }
            frame condition #1 (active) {
            }
          }
          n96 = disable-structure shown="FPGA_TARGET_CLASS==USRP_X410||FPGA_TARGET_CLASS==USRP_X410__EMBEDDED____UNSUPPORTED" {
            disable-tunnel: [refnum<k21> "RF 0/Rx/Q" ("FPGA I/O In") refnum<k21> "Daughterboard 1\\RF 1.Rx.Q2" ("FPGA I/O In")] -> w311
            disable-tunnel: [refnum<k21> "RF 0/Rx/I" ("FPGA I/O In") refnum<k21> "Daughterboard 1\\RF 1.Rx.I2" ("FPGA I/O In")] -> w312
            frame condition #0 {
            }
            frame condition #1 (active) {
            }
          }
          n97 = xnode "FPGA I/O Node"("FPGA I/O In"=w281, "FPGA I/O In"=w282) -> ("I/O Item"=w344:i16, "I/O Item"=w343:i16)  [unwired: 2 out]
          n98 = xnode "FPGA I/O Node"("FPGA I/O In"=w289, "FPGA I/O In"=w290) -> ("I/O Item"=w336:i16, "I/O Item"=w335:i16)  [unwired: 2 out]
          n99 = xnode "FPGA I/O Node"("FPGA I/O In"=w291, "FPGA I/O In"=w292) -> ("I/O Item"=w334:i16, "I/O Item"=w333:i16)  [unwired: 2 out]
          n100 = xnode "FPGA I/O Node"("FPGA I/O In"=w293, "FPGA I/O In"=w294) -> ("I/O Item"=w332:i16, "I/O Item"=w331:i16)  [unwired: 2 out]
          n101 = xnode "FPGA I/O Node"("FPGA I/O In"=w295, "FPGA I/O In"=w296) -> ("I/O Item"=w330:i16, "I/O Item"=w329:i16)  [unwired: 2 out]
          n102 = xnode "FPGA I/O Node"("FPGA I/O In"=w283, "FPGA I/O In"=w284) -> ("I/O Item"=w342:i16, "I/O Item"=w341:i16)  [unwired: 2 out]
          n103 = xnode "FPGA I/O Node"("FPGA I/O In"=w285, "FPGA I/O In"=w286) -> ("I/O Item"=w340:i16, "I/O Item"=w339:i16)  [unwired: 2 out]
          n104 = xnode "FPGA I/O Node"("FPGA I/O In"=w287, "FPGA I/O In"=w288) -> ("I/O Item"=w338:i16, "I/O Item"=w337:i16)  [unwired: 2 out]
          n105 = xnode "FPGA I/O Node"("FPGA I/O In"=w297, "FPGA I/O In"=w298) -> ("I/O Item"=w328:i16, "I/O Item"=w327:i16)  [unwired: 2 out]
          n106 = xnode "FPGA I/O Node"("FPGA I/O In"=w299, "FPGA I/O In"=w300) -> ("I/O Item"=w326:i16, "I/O Item"=w325:i16)  [unwired: 2 out]
          n107 = xnode "FPGA I/O Node"("FPGA I/O In"=w301, "FPGA I/O In"=w302) -> ("I/O Item"=w324:i16, "I/O Item"=w323:i16)  [unwired: 2 out]
          n108 = xnode "FPGA I/O Node"("FPGA I/O In"=w303, "FPGA I/O In"=w304) -> ("I/O Item"=w322:i16, "I/O Item"=w321:i16)  [unwired: 2 out]
          n109 = xnode "FPGA I/O Node"("FPGA I/O In"=w306, "FPGA I/O In"=w305) -> ("I/O Item"=w320:i16, "I/O Item"=w319:i16)  [unwired: 2 out]
          n110 = xnode "FPGA I/O Node"("FPGA I/O In"=w307, "FPGA I/O In"=w308) -> ("I/O Item"=w318:i16, "I/O Item"=w317:i16)  [unwired: 2 out]
          n111 = xnode "FPGA I/O Node"("FPGA I/O In"=w312, "FPGA I/O In"=w311) -> ("I/O Item"=w316:i16, "I/O Item"=w315:i16)  [unwired: 2 out]
          n112 = xnode "FPGA I/O Node"("FPGA I/O In"=w313, "FPGA I/O In"=w309) -> ("I/O Item"=w314:i16, "I/O Item"=w310:i16)  [unwired: 2 out]
          n113 = call-poly <instrlib>:"I16 to IQ.vi"("I"=w344, "Q"=w343) -> ("IQ"=w280:T1)  [unwired: 13 in]
          n114 = call-poly <instrlib>:"I16 to IQ.vi"("I"=w336, "Q"=w335) -> ("IQ"=w276:T1)  [unwired: 13 in]
          n115 = call-poly <instrlib>:"I16 to IQ.vi"("I"=w334, "Q"=w333) -> ("IQ"=w275:T1)  [unwired: 13 in]
          n116 = call-poly <instrlib>:"I16 to IQ.vi"("I"=w332, "Q"=w331) -> ("IQ"=w274:T1)  [unwired: 13 in]
          n117 = call-poly <instrlib>:"I16 to IQ.vi"("I"=w330, "Q"=w329) -> ("IQ"=w273:T1)  [unwired: 13 in]
          n118 = call-poly <instrlib>:"I16 to IQ.vi"("I"=w342, "Q"=w341) -> ("IQ"=w279:T1)  [unwired: 13 in]
          n119 = call-poly <instrlib>:"I16 to IQ.vi"("I"=w340, "Q"=w339) -> ("IQ"=w278:T1)  [unwired: 13 in]
          n120 = call-poly <instrlib>:"I16 to IQ.vi"("I"=w338, "Q"=w337) -> ("IQ"=w277:T1)  [unwired: 13 in]
          n121 = call-poly <instrlib>:"I16 to IQ.vi"("I"=w328, "Q"=w327) -> ("IQ"=w272:T1)  [unwired: 13 in]
          n122 = call-poly <instrlib>:"I16 to IQ.vi"("I"=w326, "Q"=w325) -> ("IQ"=w271:T1)  [unwired: 13 in]
          n123 = call-poly <instrlib>:"I16 to IQ.vi"("I"=w324, "Q"=w323) -> ("IQ"=w270:T1)  [unwired: 13 in]
          n124 = call-poly <instrlib>:"I16 to IQ.vi"("I"=w322, "Q"=w321) -> ("IQ"=w269:T1)  [unwired: 13 in]
          n125 = call-poly <instrlib>:"I16 to IQ.vi"("I"=w320, "Q"=w319) -> ("IQ"=w268:T1)  [unwired: 13 in]
          n126 = call-poly <instrlib>:"I16 to IQ.vi"("I"=w318, "Q"=w317) -> ("IQ"=w267:T1)  [unwired: 13 in]
          n127 = call-poly <instrlib>:"I16 to IQ.vi"("I"=w316, "Q"=w315) -> ("IQ"=w266:T1)  [unwired: 13 in]
          n128 = call-poly <instrlib>:"I16 to IQ.vi"("I"=w314, "Q"=w310) -> ("IQ"=w265:T1)  [unwired: 13 in]
          n129 = Build Array(w280, w279, w278, w277) -> (w264:T1[])
          n130 = Build Array(w276, w275, w274, w273) -> (w262:T1[])
          n131 = Build Array(w272, w271, w270, w269) -> (w259:T1[])
          n132 = Build Array(w268, w267, w266, w265) -> (w257:T1[])
          n133 = disable-structure shown="ACQ_CHANNEL_SWAP_0_TO_1_AND_2_TO_3==DISABLED, Default" {
            disable-tunnel: w264 -> [w348 w352]
            disable-tunnel: [w349 w352] -> w263
            disable-tunnel: w262 -> [w349 w353]
            disable-tunnel: [w348 w353] -> w261
            disable-tunnel: [w347 w351] -> w260
            disable-tunnel: w259 -> [w347 w350]
            disable-tunnel: [w346 w350] -> w258
            disable-tunnel: w257 -> [w346 w351]
            frame condition #0 (active) {
            }
            frame condition #1 {
            }
          }
          n134 = Build Array (concatenate)(w261, w263, w260, w258) -> (w345:T1[])
        }
      }
    }
  }
  "Data out" <- w1
